vi "control dc.vi"() -> ()   [LabVIEW 2019]
panel:
  in  "x":dbl
  in  "stop 5":bool
  out "ROBOT STATUS":string
  in  "START":bool
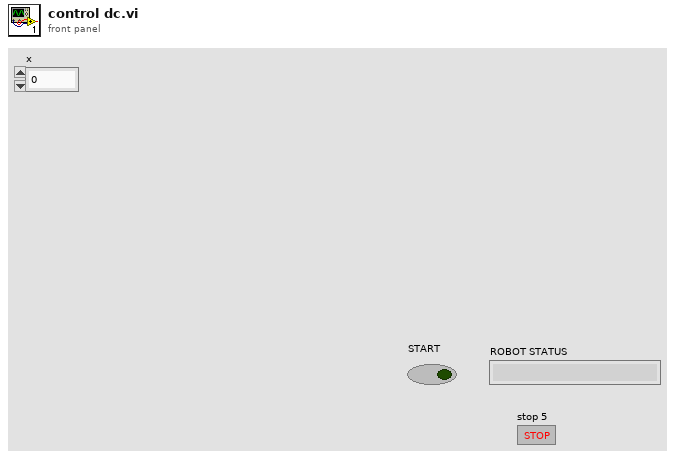
[diagram p1: front panel]
types:
  T1 = enum16{"STOP", "START", "STEP 1", "STEP 2", "STEP 3"}
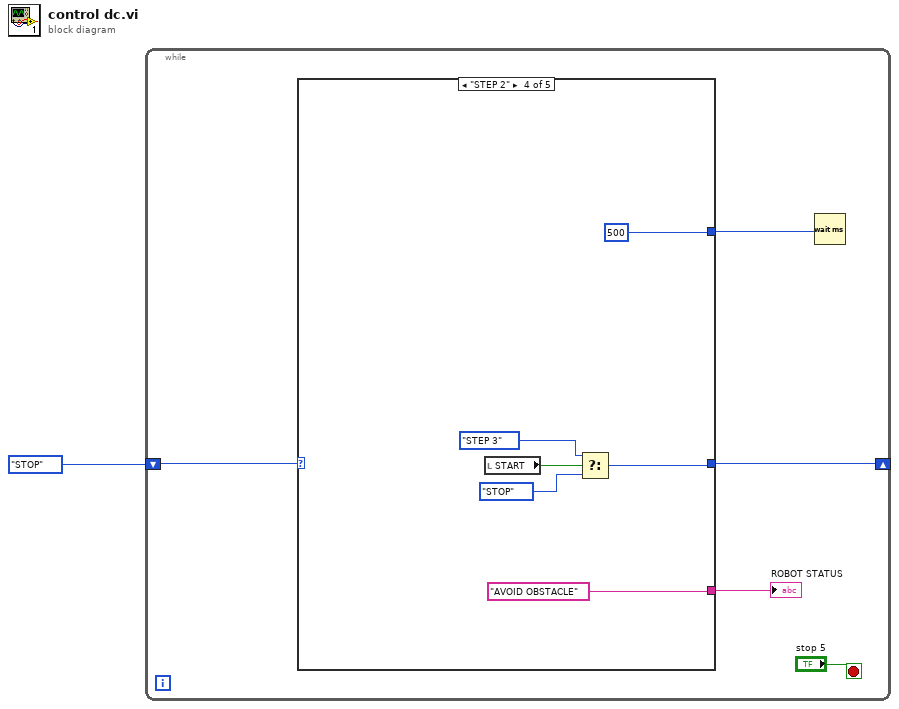
[diagram p0: block diagram]
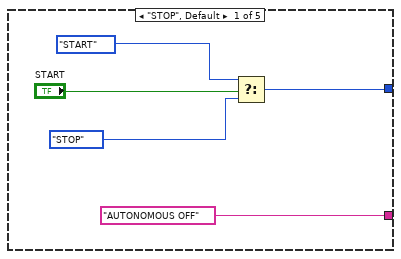
[diagram p2: hidden frame]
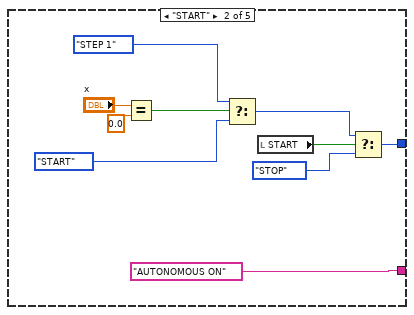
[diagram p3: hidden frame]
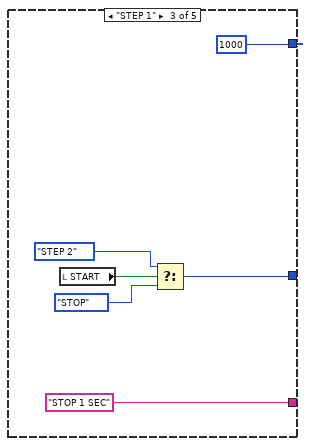
[diagram p4: hidden frame]
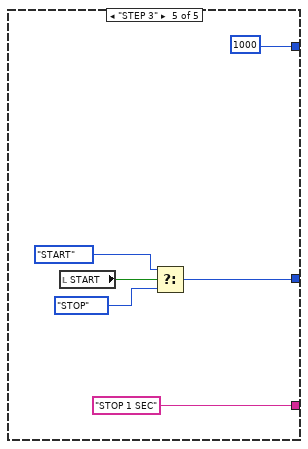
[diagram p5: hidden frame]
diagram:
  n1 = while {
    shift-right: [w4] -> _
    shift-left: T1."STOP" -> [w5]
    stop <- "stop 5" stop-if-true
    n2 = case shown="\"STEP 2\"" w5 {
      tunnel: [w9 w13 w22 w29 w35] -> w4
      tunnel: [_ _ u32 1000 ("milliseconds to wait") u32 500 ("milliseconds to wait") u32 1000 ("milliseconds to wait")] -> w3
      tunnel: ["AUTONOMOUS OFF" ("INDICATOR 4") "AUTONOMOUS ON" ("INDICATOR 4") "STOP 1 SEC" ("INDICATOR 4") "AVOID OBSTACLE" ("INDICATOR 4") "STOP 1 SEC" ("INDICATOR 4")] -> w2
      frame "STOP", Default {
        n3 = Select(t=T1."START", s="START", f=T1."STOP") -> (s? t:f=w9:T1)
      }
      frame "START" {
        n4 = Equal?(x="x", y=0.0) -> (x = y?=w20:bool)
        n5 = Select(t=T1."STEP 1", s=w20, f=T1."START") -> (s? t:f=w15:T1)
        n6 = local read "START"() -> (w16:bool)
        n7 = Select(t=w15, s=w16, f=T1."STOP") -> (s? t:f=w13:T1)
      }
      frame "STEP 1" {
        n8 = local read "START"() -> (w25:bool)
        n9 = Select(t=T1."STEP 2", s=w25, f=T1."STOP") -> (s? t:f=w22:T1)
      }
      frame "STEP 2" {
        n10 = local read "START"() -> (w32:bool)
        n11 = Select(t=T1."STEP 3", s=w32, f=T1."STOP") -> (s? t:f=w29:T1)
      }
      frame "STEP 3" {
        n12 = local read "START"() -> (w38:bool)
        n13 = Select(t=T1."START", s=w38, f=T1."STOP") -> (s? t:f=w35:T1)
      }
    }
    "ROBOT STATUS" <- w2
    n14 = Wait (ms)(milliseconds to wait=w3) -> ()  [unwired: 1 out]
  }
